vi "Sub_Pin_Torsion.vi"(9 "Torsion":dbl, 10 "Pin Location":i32, 11 "K Matrix Input":dbl[][](array[numeric])) -> (3 "K Matrix Output":dbl[][](array[numeric]))   [LabVIEW 2021]
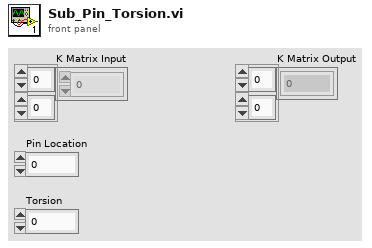
[diagram p1: front panel]
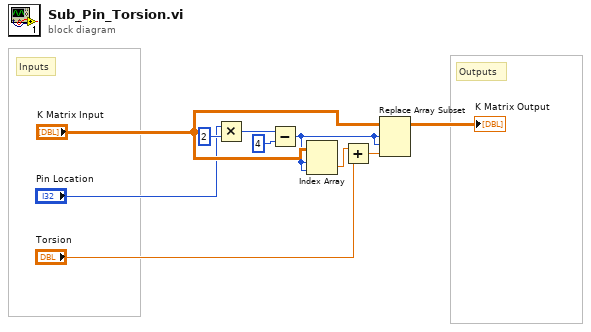
[diagram p0: block diagram]
diagram:
  # "Outputs"
  # "Inputs"
  n1 = Multiply(x="Pin Location", y=2) -> (x*y=w3:i32)
  n2 = Subtract(x=w3, y=4) -> (x-y=w1:i32)
  n3 = Index Array(array="K Matrix Input", index (row)=w1, index (col)=w1) -> (element=w7:dbl)
  n4 = Add(x=w7, y="Torsion") -> (x+y=w10:dbl)
  n5 = Replace Array Subset(array="K Matrix Input", new element=w10, index (row)=w1, index (col)=w1) -> (→"K Matrix Output":dbl[][])
